vi "Hide Panel.vi"(8 "error in (no error)":errorcluster, 10 "Panel":refnum<class "Panel.lvclass">, 11 "PanelManager in":refnum<class "PanelManager.lvclass">) -> (0 "error out":errorcluster, 3 "PanelManager out":refnum<class "PanelManager.lvclass">)   [LabVIEW 2018, in "OOPanel.lvlib" / "PanelManager.lvclass"]
uses:
  PanelManager.lvclass
  Panel/Panel.lvclass
  Panel/State.ctl
  PanelManager.lvclass/PanelManager.ctl
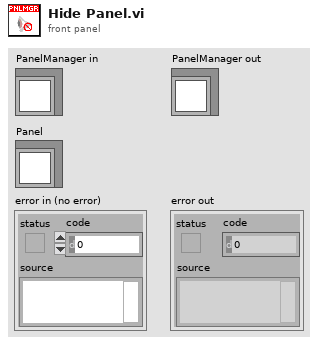
[diagram p1: front panel]
types:
  T1 = typedef "OOPanel.lvlib/Panel.lvclass/State.ctl" = enum16{"Idle", "Hidden", "Visible", "Subpanel"}
  T2 = enum32{"Invalid", "Standard", "Closed", "Hidden", "Minimized", "Maximized"}
  T3 = typedef "OOPanel.lvlib/PanelManager.lvclass/Ref Data.ctl" = cluster{"Panels":T4, "Subpanel Map":T5}
  T4 = typedef "OOPanel.lvlib/PanelManager.lvclass/Panels.ctl" = cluster{"Names":string[], "Instances":refnum<class "Panel.lvclass">[]}
  T5 = typedef "OOPanel.lvlib/PanelManager.lvclass/SubPanel Map.ctl" = cluster{"SubPanels":refnum<vi>[], "Panels":refnum<class "Panel.lvclass">[]}
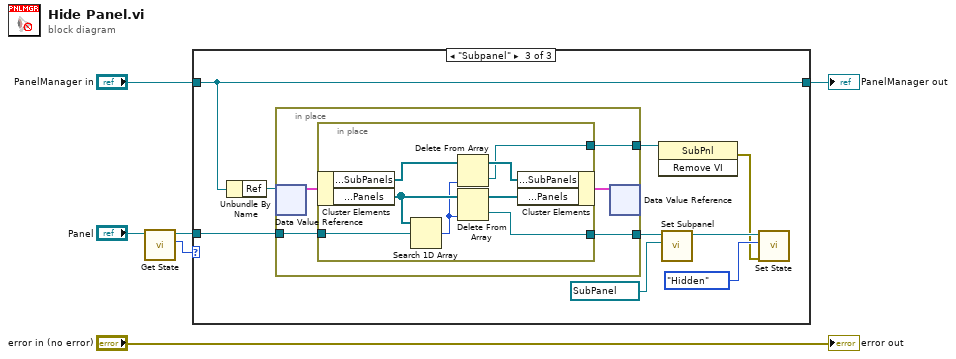
[diagram p0: block diagram]
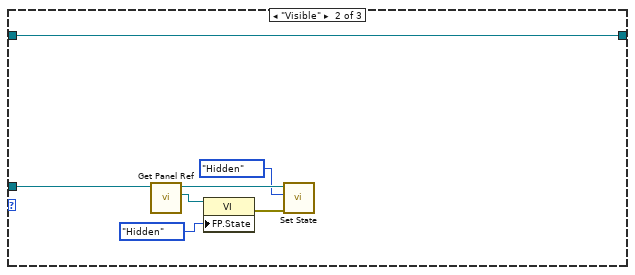
[diagram p3: hidden frame]
diagram:
  n1 = call "Get State.vi"("Panel in"="Panel") -> ("State"=w3:T1, "Panel out"=w5:refnum<class "Panel.lvclass">)  [unwired: 8 in, 1 out]
  n2 = case shown="\"Subpanel\"" w3 {
    tunnel: w5 -> [_ w12 w21]
    tunnel: "PanelManager in" -> [w7 w11 w22]
    tunnel: [w7 w11 w22] -> w1
    frame Default {
    }
    frame "Visible" {
      n3 = call "Get Panel Ref.vi"("Panel in"=w12) -> ("Panel Ref"=w14:refnum<vi>, "Panel out"=w10:refnum<class "Panel.lvclass">)  [unwired: 8 in, 1 out]
      n4 = property class="VI"(reference=w14, "FP.State"=T2."Hidden" ("Front Panel Window:State")) -> (error out=w9:errorcluster)  [unwired: 1 in, 1 out]
      n5 = call "Set State.vi"("error in (no error)"=w9, "State"=State."Hidden", "Panel in"=w10) -> ()  [unwired: 7 in, 2 out]
    }
    frame "Subpanel" {
      n6 = Unbundle By Name(w22) -> ("Ref"=w23:refnum<data-value>)
      n7 = in-place {
        in-place-border: w21 -> [w26]
        in-place-border: [w25] -> w19
        in-place-border: [w24] -> w20
        n8 = in-place-dvr #1(w23) -> (w28:T3)  [unwired: 1 out]
        n9 = in-place {
          in-place-border: w26 -> [w36]
          in-place-border: [w30] -> w25
          in-place-border: [w29] -> w24
          n10 = in-place-cluster #2(w28) -> ("Subpanel Map.SubPanels"=w34:refnum<vi>[], "Subpanel Map.Panels"=w35:refnum<class "Panel.lvclass">[])
          n11 = Search 1D Array(1D array=w35, element=w36) -> (index of element=w31:i32)  [unwired: 1 in]
          n12 = Delete From Array(array=w34, index=w31) -> (deleted portion=w29:refnum<vi>, array with subset deleted=w33:refnum<vi>[])  [unwired: 1 in]
          n13 = Delete From Array(array=w35, index=w31) -> (deleted portion=w30:refnum<class "Panel.lvclass">, array with subset deleted=w32:refnum<class "Panel.lvclass">[])  [unwired: 1 in]
          n14 = in-place-cluster #2("Subpanel Map.SubPanels"=w33, "Subpanel Map.Panels"=w32) -> (w27:T3)
        }
        n15 = in-place-dvr #1(w27) -> ()  [unwired: 2 out]
      }
      n16 = invoke class="SubPnl" method="Remove VI"(reference=w20) -> (error out=w15:errorcluster)  [unwired: 2 in, 2 out]
      n17 = call "Set Subpanel.vi"("Subpanel"=refnum<vi> refnum, "Panel in"=w19) -> ("Panel out"=w16:refnum<class "Panel.lvclass">)  [unwired: 8 in, 1 out]
      n18 = call "Set State.vi"("error in (no error)"=w15, "State"=State."Hidden", "Panel in"=w16) -> ()  [unwired: 7 in, 2 out]
    }
  }
  "PanelManager out" <- w1
  "error out" <- "error in (no error)"
